vi "Gestion_TAGs_ARAbia.vi"() -> ()   [LabVIEW 2015]
panel:
  out "Array 2":string[](array[string])
  out "Array":string[][](array[string])
  out "x = y?":bool
  in  "Tags_desorden":string[](array[string])
  out "Ejes_convoy":i32
  out "Nº Ejes":i32[](array[numeric])
  out "Nº UTs":i32
  in  "Tabla_flota":string[][](array[string])=[["Flota", "UT", "Ejes", "Tag inicio", "Tag fin"], ["MB", "501", "10", "2003480000000000000001F5", "0000000A00000000000001F5"], ["MB", "502", "12", "2003480000000000000001F6", "0000000A00000000000001F6"], ["MB", "503", "15", "2003480000000000000001F7", "0000000A00000000000001F7"], ["MB", "504", "19", "2003480000000000000001F8", "0000000A00000000000001F8"], ["MB", "505", "23", "2003480000000000000001F9", "0000000A00000000000001F9"]]
  out "TAGs ordenados 2":string[](array[string])
  out "Plataformas?":bool
  out "TAGs_ ordenados_1":i32[](array[numeric])
  out "TAGs ordenados_1":string[](array[string])
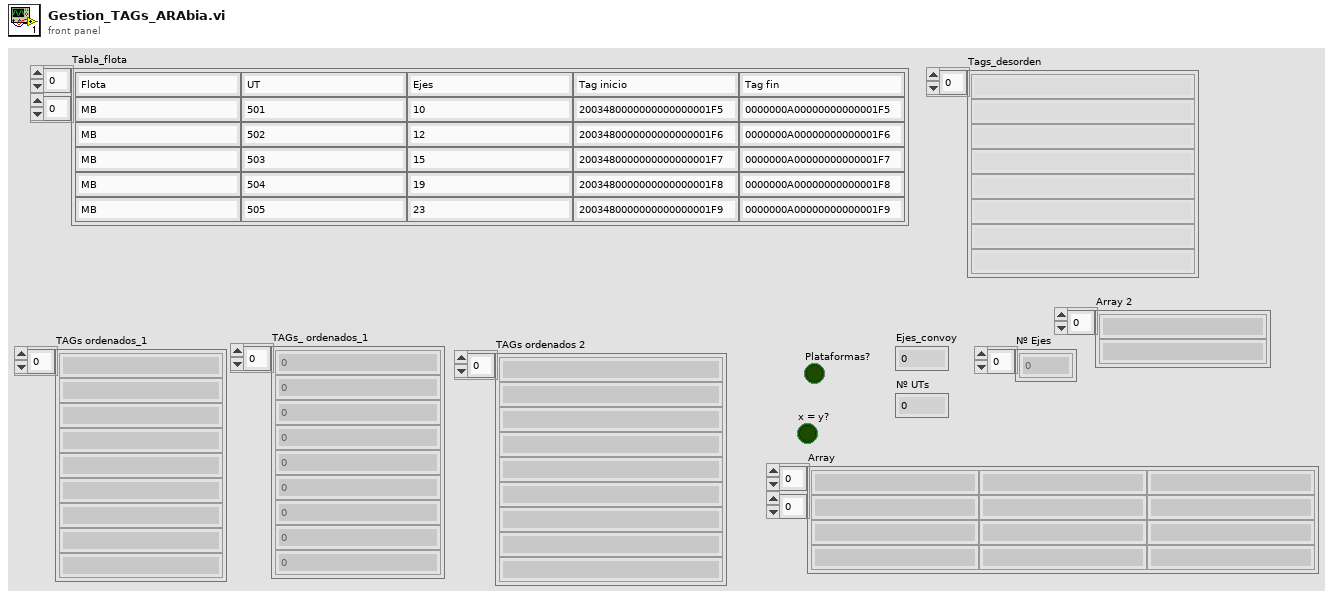
[diagram p1: front panel]
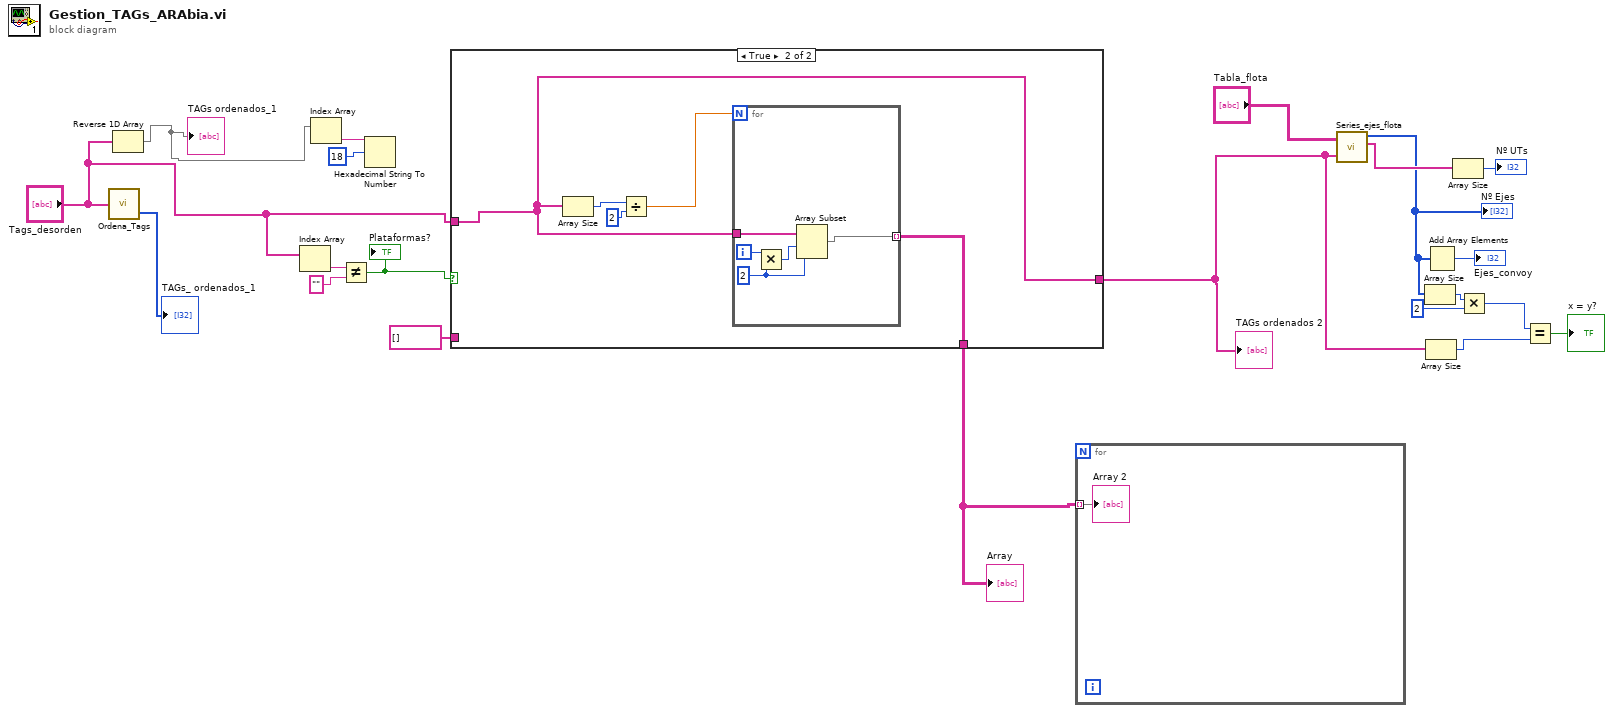
[diagram p0: block diagram]
diagram:
  n1 = call "Ordena_Tags.vi"("Tags_desorden"="Tags_desorden") -> ("sorted array"=→"TAGs_ ordenados_1":i32[])  [unwired: 1 out]
  n2 = Reverse 1D Array(array="Tags_desorden") -> (reversed array=w10:string[])
  "TAGs ordenados_1" <- w10
  n3 = Index Array(array="Tags_desorden") -> (element=w18:string)  [unwired: 1 in]
  n4 = Index Array(array=w10) -> (element=w20:string)  [unwired: 1 in]
  n5 = Not Equal?(x=w18, y="" ("delimiter (\\t)")) -> (x != y?=w16:bool)
  "Plataformas?" <- w16
  n6 = Hexadecimal String To Number(string=w20, offset=18) -> ()  [unwired: 3 out]
  n7 = case shown="True" w16 {
    tunnel: string[] [] -> [w22 _]
    tunnel: [w22 w24] -> w6
    tunnel: "Tags_desorden" -> [_ w24]
    tunnel: [_ w23] -> w1
    frame False {
    }
    frame True {
      n8 = Array Size(array=w24) -> (size(s)=w27:i32)
      n9 = Divide(x=w27, y=2) -> (x/y=w25:dbl)
      n10 = for {
        N: w25 -> [_]
        tunnel: w24 -> [w32]
        tunnel: [w28] -> w23 mode=indexing
        i -> [w31]
        w29 = 2 ("y")
        n11 = Multiply(x=w31, y=w29) -> (x*y=w30:i32)
        n12 = Array Subset(array=w32, index=w30, length=w29) -> (w28:string[])
      }
    }
  }
  "TAGs ordenados 2" <- w6
  "Array" <- w1
  n13 = for {
    tunnel: w1 -> [w33] mode=indexing
    "Array 2" <- w33
  }
  n14 = call "Series_ejes_flota.vi"("Tabla_flota"="Tabla_flota", "Tags"=w6) -> ("Nº Ejes"=w9:i32[], "Series del convoy"=w11:string[])  [unwired: 2 in, 1 out]
  "Nº Ejes" <- w9
  n15 = Array Size(array=w9) -> (size(s)=w8:i32)
  n16 = Array Size(array=w6) -> (size(s)=w4:i32)
  n17 = Add Array Elements(numeric array=w9) -> (sum=→"Ejes_convoy":i32)
  n18 = Array Size(array=w11) -> (size(s)=→"Nº UTs":i32)
  n19 = Multiply(x=w8, y=2) -> (x*y=w5:i32)
  n20 = Equal?(x=w5, y=w4) -> (x = y?=→"x = y?":bool)
